vi "Bind Boolean Text.vi"(4 "Ignore Past Updates? (F)":bool, 5 "Datum Type":variant, 6 "Format String":string, 8 "error in (no error)":errorcluster, 9 "Datum Name (\"\"=Use Control Label)":string, 10 "Bool Refnum":refnum<vi>, 11 "IViewable in":refnum<class "IViewable.lvclass">) -> (0 "error out":errorcluster, 3 "IViewable out":refnum<class "IViewable.lvclass">)   [LabVIEW 2020, in "IViewable.lvlib" / "IViewable.lvclass"]
uses:
  <vilib>/gpm_packages/@cs/mva-viewable/Source/IViewable/IViewable/IViewable.lvclass
  C:/Program Files/National Instruments/LabVIEW 2020/vi.lib/ActorFramework/Actor/Actor.lvclass
  <vilib>/ActorFramework/Actor/Actor.lvclass/Actor.ctl
  <vilib>/ActorFramework/Message Enqueuer/Message Enqueuer.lvclass/Message Enqueuer.ctl
  <vilib>/gpm_packages/@cs/mva-core/Source/SubscriptionPolicy/ValueChangeSubscription/ValueChangeSubscription.lvclass/ValueChangeSubscription.ctl
  <vilib>/gpm_packages/@cs/transport/Source/Concrete/BooleanTextBinding/BooleanTextBinding.lvclass/BooleanTextBinding.ctl
  <vilib>/gpm_packages/@cs/mva-core/Source/IMediator/SubscriptionRequest/SubscriptionRequest.lvclass/SubscriptionRequest.ctl
  <vilib>/gpm_packages/@cs/mva-core/Source/IObserver/IObserver Messages/Subscribe Msg/Subscribe Msg.lvclass/Subscribe Msg.ctl
  <vilib>/ActorFramework/Message Enqueuer/Enqueue.vi
  <vilib>/ActorFramework/Message Enqueuer/Init from Existing Queue.vi
  <vilib>/gpm_packages/@cs/mva-core/Source/SubscriptionPolicy/ValueChangeSubscription/ValueChangeSubscription.lvclass
  C:/Program Files/National Instruments/LabVIEW 2020/vi.lib/gpm_packages/@cs/mva-core/Source/IMediator/ISubscriptionPolicy/ISubscriptionPolicy.lvclass
  <vilib>/gpm_packages/@cs/transport/Source/Concrete/BooleanTextBinding/BooleanTextBinding.lvclass
  C:/Program Files/National Instruments/LabVIEW 2020/vi.lib/gpm_packages/@cs/transport/Source/ITransport/ITransport.lvclass
  <vilib>/gpm_packages/@cs/mva-core/Source/IObserver/IObserver Messages/Subscribe Msg/Subscribe Msg.lvclass
  C:/Program Files/National Instruments/LabVIEW 2020/vi.lib/ActorFramework/Message/Message.lvclass
  <vilib>/Utility/error.llb/Error Cluster From Error Code.vi
  <vilib>/ActorFramework/Message Priority Queue/Priority Enqueue.vi
  <vilib>/gpm_packages/@cs/mva-core/Source/IMediator/SubscriptionRequest/SubscriptionRequest.lvclass
  <vilib>/ActorFramework/Message Enqueuer/Message Enqueuer.lvclass
  <vilib>/ActorFramework/Actor/Actor.lvclass
  <vilib>/gpm_packages/@cs/mva-core/Source/IMediator/ISubscriptionPolicy/ISubscriptionPolicy.lvclass
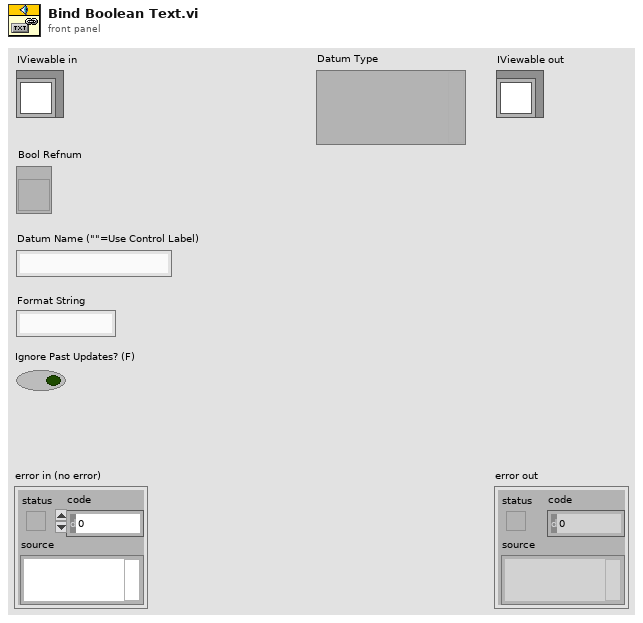
[diagram p1: front panel]
types:
  T1 = typedef "IMediator.lvlib/ISubscriptionPolicy.lvclass/ISubscriptionPolicy Reference.ctl" = refnum<data-value>
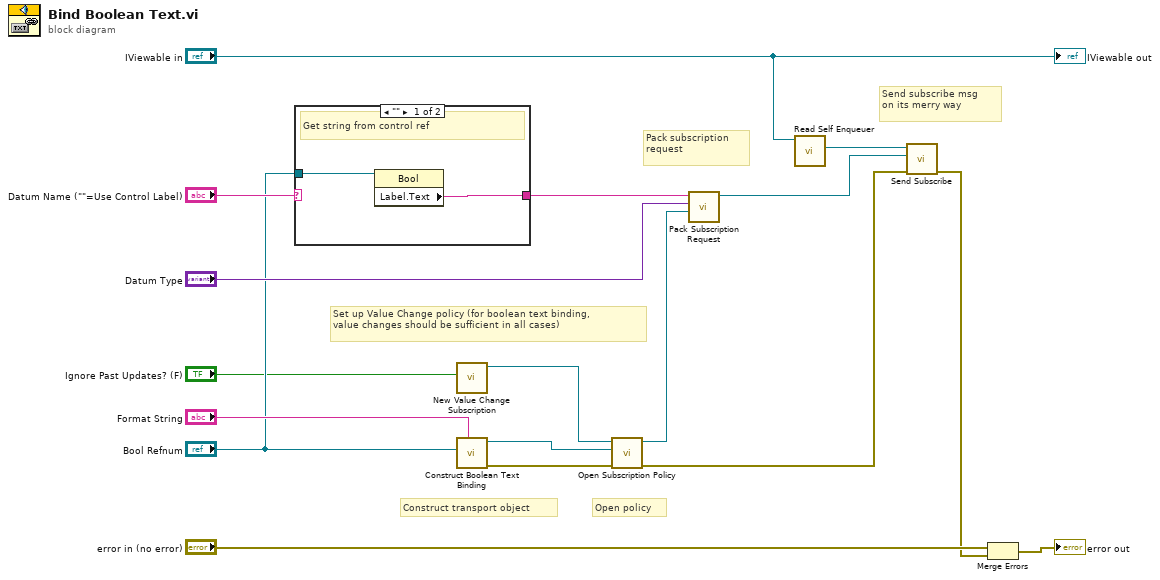
[diagram p0: block diagram]
diagram:
  # "Open policy"
  # "Set up Value Change policy (for boolean text binding,\nvalue changes should be sufficient in all cases)"
  # "Send subscribe msg\non its merry way"
  # "Pack subscription\nrequest"
  # "Construct transport object"
  n1 = case shown="\"\"" "Datum Name (\"\"=Use Control Label)" {
    selector: "Datum Name (\"\"=Use Control Label)" -> [_ w20]
    tunnel: [w18 w20] -> w11
    tunnel: "Bool Refnum" -> [w19 _]
    frame "" {
      # "Get string from control ref"
      n2 = property class="Bool"(reference=w19) -> ("Label.Text"=w18:string)  [unwired: 1 in, 2 out]
    }
    frame Default {
      # "Use string wired to input terminal"
    }
  }
  n3 = call <vilib>:"New Value Change Subscription.vi"("Ignore Past Updates? (F)"="Ignore Past Updates? (F)") -> ("ValueChangeSubscription Out"=w4:refnum<class "ValueChangeSubscription.lvclass">)  [unwired: 10 in]
  n4 = call <vilib>:"Construct Boolean Text Binding.vi"("Format String"="Format String", "Bool Refnum"="Bool Refnum") -> ("error out"=w2:errorcluster, "BooleanTextBinding"=w7:refnum<class "BooleanTextBinding.lvclass">)  [unwired: 8 in]
  n5 = call <vilib>:"Open Subscription Policy.vi"("error in (no error)"=w2, "Transport"=w7, "SubscriptionPolicy"=w4) -> ("error out"=w1:errorcluster, "Subscription Policy"=w3:T1)  [unwired: 7 in]
  n6 = call <vilib>:"Pack Subscription Request.vi"("Subscription Policy"=w3, "Type"="Datum Type", "Datum Name"=w11) -> ("SubscriptionRequest"=w6:refnum<class "SubscriptionRequest.lvclass">)  [unwired: 7 in, 1 out]
  n7 = call <vilib>:"Read Self Enqueuer.vi"("Actor"="IViewable in") -> ("Self Enqueuer"=w15:refnum<class "Message Enqueuer.lvclass">)  [unwired: 10 in]
  n8 = call <vilib>:"Send Subscribe.vi"("error in (no error)"=w1, "SubscriptionRequest"=w6, "Message Enqueuer"=w15) -> ("error out"=w13:errorcluster)  [unwired: 7 in, 1 out]
  n9 = Merge Errors("error in (no error)", w13) -> (→"error out":errorcluster)
  "IViewable out" <- "IViewable in"
